vi "Subscribe Actor to Class Topic.vi"(4 "Excluded (None)":refnum<class "Message.lvclass">[](array[class]), 5 "Channel Class":refnum<class "Pub Sub Message Channel.lvclass">, 6 "Included (All)":refnum<class "Message.lvclass">[](array[class]), 8 "error in (no error)":errorcluster, 9 "Name":string, 10 "Receivers Enqueuer":refnum<class "Message Enqueuer.lvclass">, 11 "Topic":refnum<class>) -> (0 "error out":errorcluster, 3 "Channel Out":refnum<class "Pub Sub Message Channel.lvclass">)   [LabVIEW 2020, in "Actor Pub Sub Channels.lvlib"]
uses:
  Actor Pub Sub Channels.lvlib
  <vilib>/ActorFramework/Message Enqueuer/Message Enqueuer.lvclass
  Pub Sub Message Channel/Pub Sub Message Channel.lvclass
  <vilib>/ActorFramework/Message/Message.lvclass
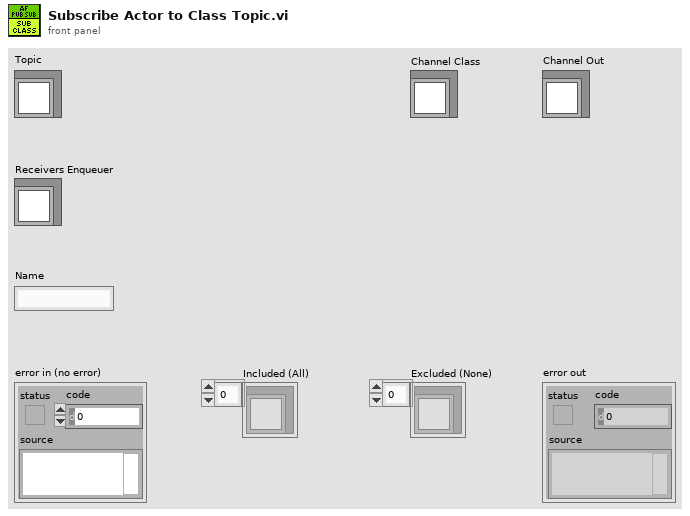
[diagram p1: front panel]
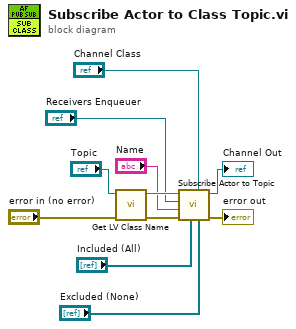
[diagram p0: block diagram]
diagram:
  n1 = call <vilib>:"Get LV Class Name.vi"("error in (no error)"="error in (no error)", "object"="Topic") -> ("error out"=w9:errorcluster, "class name"=w8:string)  [unwired: 8 in]
  n2 = call "Subscribe Actor to Topic.vi"("Excluded (None)"="Excluded (None)", "Channel Class"="Channel Class", "Included (All)"="Included (All)", "error in (no error)"=w9, "Name"="Name", "Receivers Enqueuer"="Receivers Enqueuer", "Topic"=w8) -> ("error out"=→"error out":errorcluster, "Channel Out"=→"Channel Out":refnum<class "Pub Sub Message Channel.lvclass">)  [unwired: 2 in, 1 out]
